vi "AcquisitionPlay.vi"(0 "task/channels in":refnum<k21>, 7 "number of samples per channel":i32=-1, 11 "error in":errorcluster) -> (4 "task out":refnum<k21>, 8 "data":waveform(dbl)[](array[waveform]), 15 "error out":errorcluster)   [LabVIEW 2025]
uses:
  <vilib>/DAQmx/read.llb/DAQmx Read (Analog 1D Wfm NChan NSamp).vi
  <vilib>/DAQmx/miscellaneous.llb/DAQmx Fill In Error Info.vi
panel:
  # "Inicia la adquisición de datos"
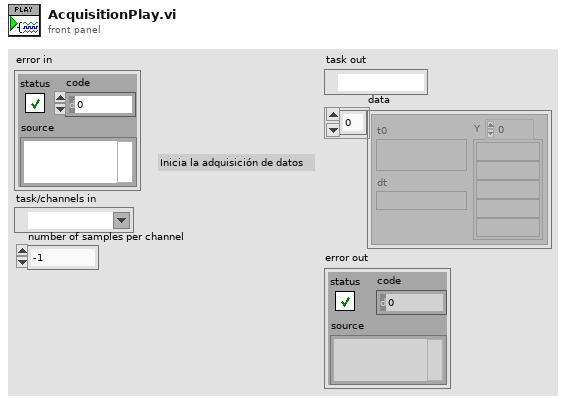
[diagram p1: front panel]
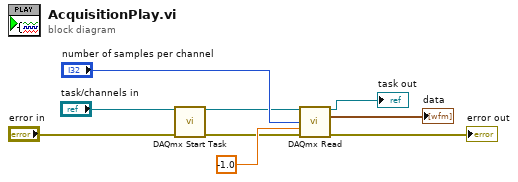
[diagram p0: block diagram]
diagram:
  n1 = call <vilib>:"DAQmx Start Task.vi"("task/channels in"="task/channels in", "error in"="error in") -> ("task out"=w5:refnum<k21>, "error out"=w4:errorcluster)  [unwired: 12 in]
  n2 = call-poly <vilib>:"DAQmx Read.vi"("task/channels in"=w5, "number of samples per channel"="number of samples per channel", "timeout"=-1.0, "error in"=w4) -> ("task out"=→"task out":refnum<k21>, "data"=→"data":waveform(dbl)[], "error out"=→"error out":errorcluster)  [unwired: 9 in]
